vi "Set RTB Selection Text Background Color.vi"(8 "Error In":errorcluster, 9 "Text Background Color":T1=enum."Black", 11 ".NET RTB Refnum in":refnum<k24>) -> (0 "Error Out":errorcluster, 3 ".NET RTB Refnum out":refnum<k24>)   [LabVIEW 2019, in "Rich Text Box.lvlib"]
uses:
  Rich Text Box.lvlib
  Text Colors.ctl
  System.Windows.Forms
  System.Drawing
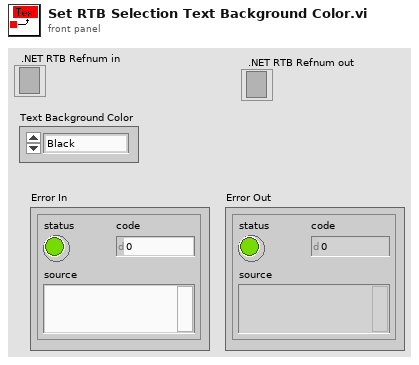
[diagram p1: front panel]
types:
  T1 = typedef "Rich Text Box.lvlib/Text Colors.ctl" = enum16{"Unchanged", "Black", "Blue", "Gray", "Green", "Red", "White"}
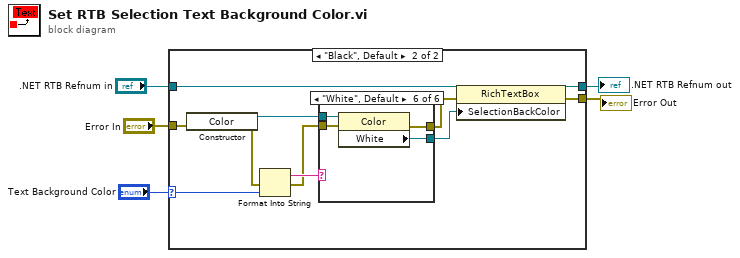
[diagram p0: block diagram]
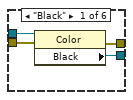
[diagram p3: hidden frame]
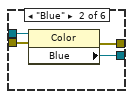
[diagram p4: hidden frame]
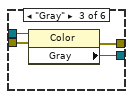
[diagram p5: hidden frame]
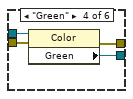
[diagram p6: hidden frame]
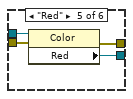
[diagram p7: hidden frame]
diagram:
  n1 = case shown="\"Black\", Default" "Text Background Color" {
    selector: "Text Background Color" -> [_ w14]
    tunnel: ".NET RTB Refnum in" -> [w7 w16]
    tunnel: [w7 w12] -> w3
    tunnel: [w6 w11] -> w2
    tunnel: "Error In" -> [w6 w10]
    frame "Unchanged" {
    }
    frame "Black", Default {
      n2 = constructor class="Color"(error in=w10) -> (reference out=w15:refnum<k24>, error out=w9:errorcluster)  [unwired: 2 in, 1 out]
      n3 = Format Into String(error in=w9, w14) -> (resulting string=w13:string, error out=w8:errorcluster)  [unwired: 2 in]
      n4 = case shown="\"White\", Default" w13 {
        tunnel: w15 -> [w22 w26 w30 w34 w38 w42]
        tunnel: w8 -> [w21 w25 w29 w33 w37 w41]
        tunnel: [w20 w24 w28 w32 w36 w40] -> w17
        tunnel: [w19 w23 w27 w31 w35 w39] -> w18
        frame "Black" {
          n5 = property class="Color"(reference=w22, error in=w21) -> (error out=w19:errorcluster, "Black"=w20:refnum<k24>)  [unwired: 1 out]
        }
        frame "Blue" {
          n6 = property class="Color"(reference=w26, error in=w25) -> (error out=w23:errorcluster, "Blue"=w24:refnum<k24>)  [unwired: 1 out]
        }
        frame "Gray" {
          n7 = property class="Color"(reference=w30, error in=w29) -> (error out=w27:errorcluster, "Gray"=w28:refnum<k24>)  [unwired: 1 out]
        }
        frame "Green" {
          n8 = property class="Color"(reference=w34, error in=w33) -> (error out=w31:errorcluster, "Green"=w32:refnum<k24>)  [unwired: 1 out]
        }
        frame "Red" {
          n9 = property class="Color"(reference=w38, error in=w37) -> (error out=w35:errorcluster, "Red"=w36:refnum<k24>)  [unwired: 1 out]
        }
        frame "White", Default {
          n10 = property class="Color"(reference=w42, error in=w41) -> (error out=w39:errorcluster, "White"=w40:refnum<k24>)  [unwired: 1 out]
        }
      }
      n11 = property class="RichTextBox"(reference=w16, error in=w18, "SelectionBackColor"=w17) -> (reference out=w12:refnum<k24>, error out=w11:errorcluster)
    }
  }
  ".NET RTB Refnum out" <- w3
  "Error Out" <- w2
